vi "Dot product_3Dpf.vi"(1 "B":sgl[](array[numeric]), 2 "A":sgl[](array[numeric])) -> (0 "A . B":sgl)   [LabVIEW 2017]
panel:
  # "PN 12/01/2015"
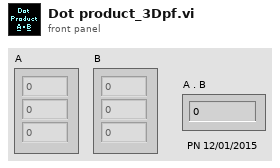
[diagram p1: front panel]
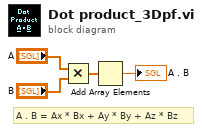
[diagram p0: block diagram]
diagram:
  # "A . B = Ax * Bx + Ay * By + Az * Bz"
  n1 = Multiply(x="A", y="B") -> (x*y=w2:sgl[])
  n2 = Add Array Elements(numeric array=w2) -> (sum=→"A . B":sgl)
